vi "Configure IQ Recorder Measurement Parameters.vi"(6 "File Path (\"C:\\Temp\\IQRecorder\\Results\\IQSaveFile.txt\")":string="C:\\Temp\\IQRecorder\\Results\\IQSaveFile.txt", 7 "Samples After (512)":i32=512, 8 "error in (no error)":errorcluster, 9 "Samples Before (512)":i32=512, 10 "Instance (1)":i32=1 format="%.0g", 11 "VISA resource name":refnum<visa-resource-name>) -> (0 "error out":errorcluster, 3 "VISA resource name out":refnum<visa-resource-name>)   [LabVIEW 2015, in "Rohde&Schwarz CMXP GPRF.lvlib"]
doc: "Configures IQ Recorder measurement parameters.\n\nAttribute:\nRSCMXPGPRF_ATTR_IQ_RECORDER_FILE_PATH\n\nRemote-control commands:\nCONFigure:GPRF:MEAS<i>:IQRecorder:CAPTure\nCONFigure:GPRF:MEAS<i>:IQRecorder:IQFile"
uses:
  <instrlib>/Rohde&Schwarz CMXP GPRF/Rohde&Schwarz CMXP GPRF.lvlib
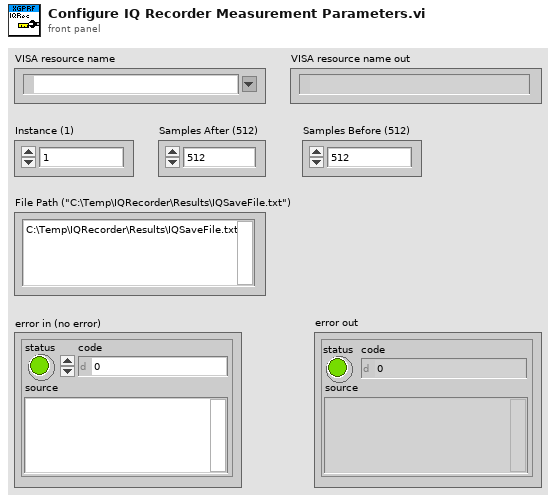
[diagram p1: front panel]
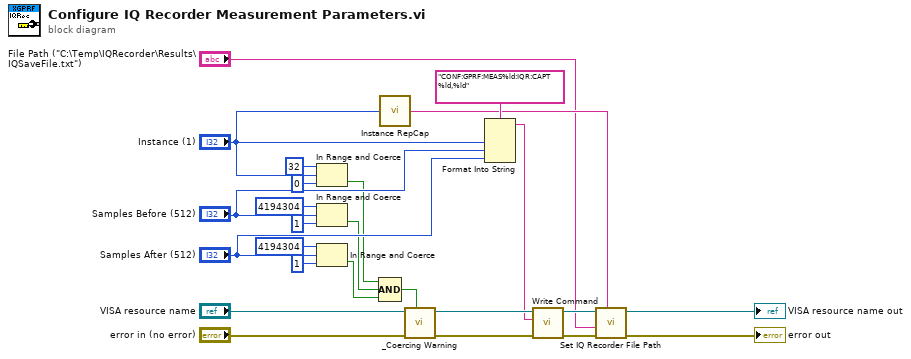
[diagram p0: block diagram]
diagram:
  n1 = In Range and Coerce(upper limit=32, x="Instance (1)", lower limit=0) -> (In Range?=w3:bool)  [unwired: 1 out]
  n2 = In Range and Coerce(upper limit=4194304, x="Samples Before (512)", lower limit=1) -> (In Range?=w4:bool)  [unwired: 1 out]
  n3 = In Range and Coerce(upper limit=4194304, x="Samples After (512)", lower limit=1) -> (In Range?=w5:bool)  [unwired: 1 out]
  n4 = Compound Arithmetic op=AND(w3, w4, w5) -> (w8:bool)
  n5 = call <instrlib>:"Instance RepCap.vi"("instance  in"="Instance (1)") -> ("instance out"=w17:string)
  n6 = call <instrlib>:"_Coercing Warning.vi"("In Range?"=w8, "error in (no error)"="error in (no error)", "VISA resource name"="VISA resource name") -> ("error out"=w21:errorcluster, "VISA resource name out"=w22:refnum<visa-resource-name>)  [unwired: 7 in]
  n7 = Format Into String(format string="CONF:GPRF:MEAS%ld:IQR:CAPT %ld,%ld", "Instance (1)", "Samples Before (512)", "Samples After (512)") -> (resulting string=w1:string)  [unwired: 2 in, 1 out]
  n8 = call <instrlib>:"Write Command.vi"("error in (no error)"=w21, "Command"=w1, "VISA resource name"=w22) -> ("error out"=w15:errorcluster, "VISA resource name out"=w16:refnum<visa-resource-name>)  [unwired: 7 in]
  n9 = call "Set IQ Recorder File Path"("Repeated Capabilities"=w17, "error in (no error)"=w15, "IQ Recorder File Path ()"="File Path (\"C:\\Temp\\IQRecorder\\Results\\IQSaveFile.txt\")", "instrument handle"=w16) -> ("error out"=→"error out":errorcluster, "instrument handle out"=→"VISA resource name out":refnum<visa-resource-name>)  [unwired: 6 in]
